vi "Main.vi"() -> ()   [LabVIEW 2015]
doc: "Use this template to build a simple state machine design pattern. Each state executes code and determines which state to transition to."
uses:
  controls/State.ctl
  controls/Data.ctl
  <vilib>/measure/NI_MABase.lvlib
panel:
  in  "Dateiname":string
  out "Waveform Chart":waveform(dbl)(graph)
  in  "Daten speichern":bool
  in  "Signal generieren":bool
  in  "Exit":bool
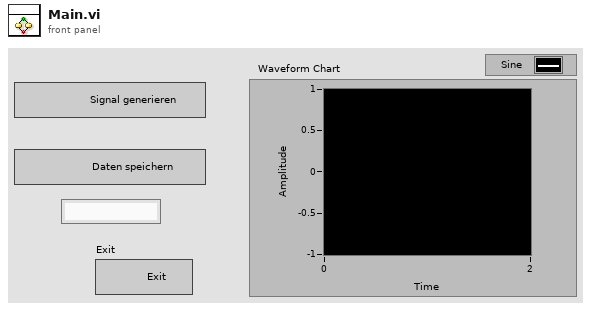
[diagram p1: front panel]
types:
  T1 = typedef "Data.ctl" = cluster{"Boolean":bool, "String":string, "Numeric":dbl, "Waveform":waveform(dbl)}
  T2 = typedef "State.ctl" = enum16{"Initialize", "Wait for Event", "Signal generieren", "Daten speichern", "Exit"}
  T3 = enum16{"open", "open or create", "create or replace", "create", "open (read-only)"}
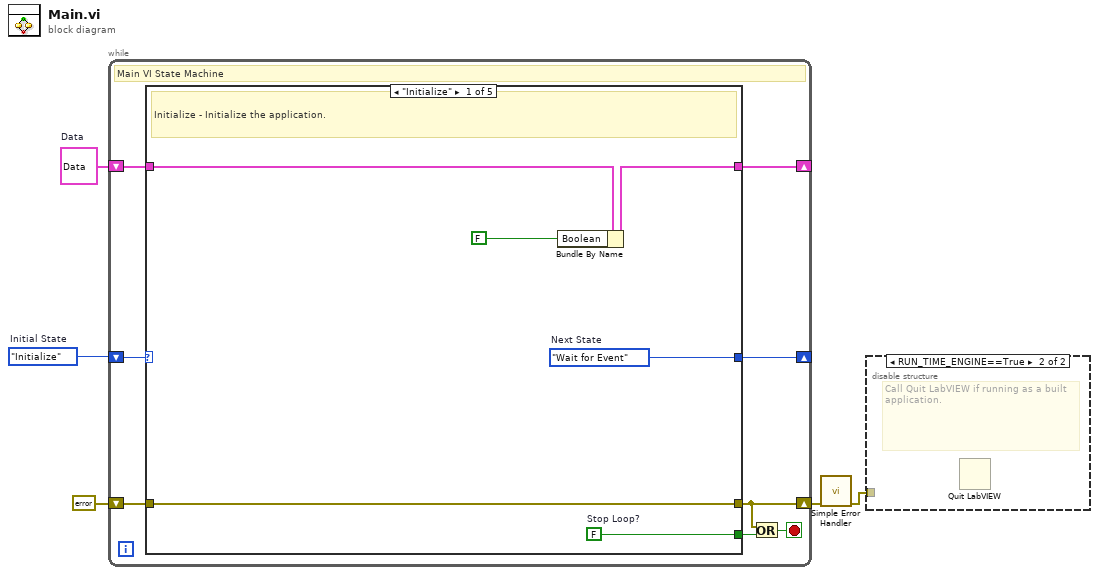
[diagram p0: block diagram]
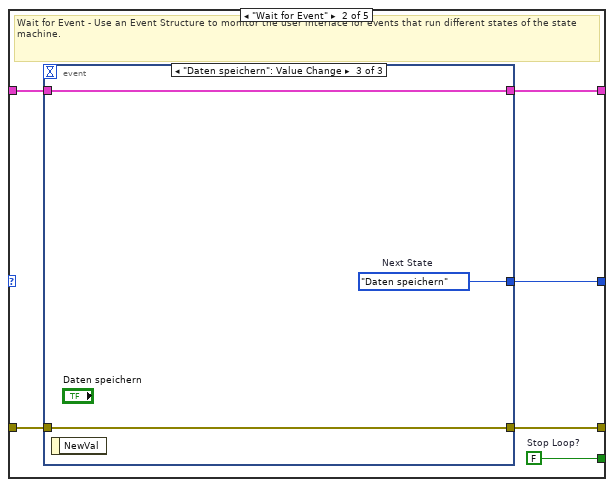
[diagram p3: hidden frame]
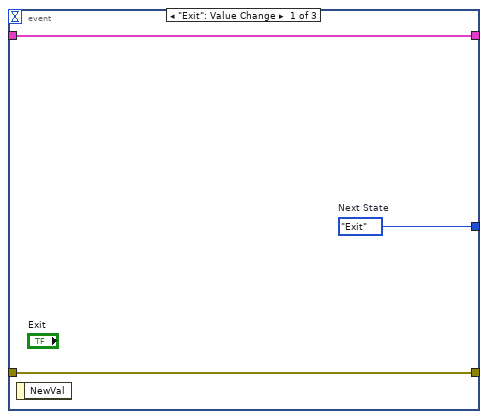
[diagram p4: hidden frame]
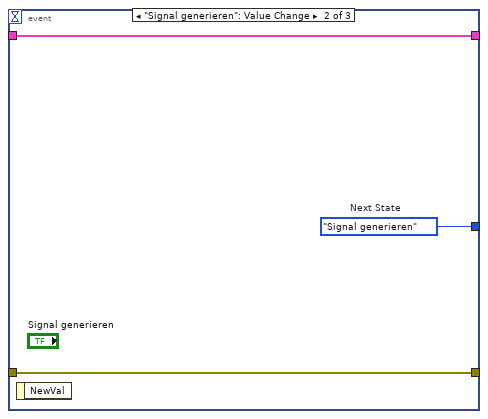
[diagram p5: hidden frame]
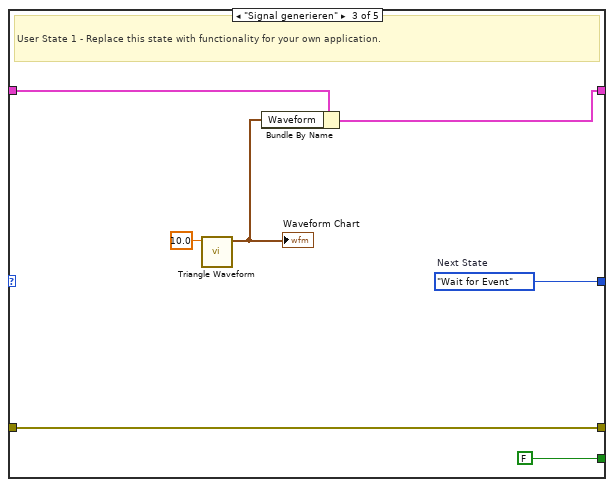
[diagram p6: hidden frame]
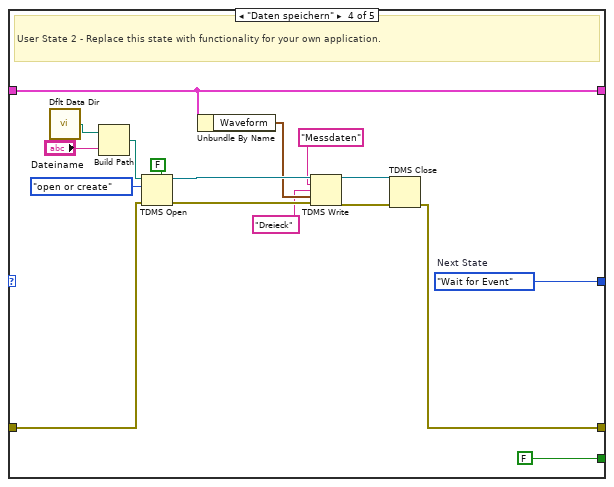
[diagram p7: hidden frame]
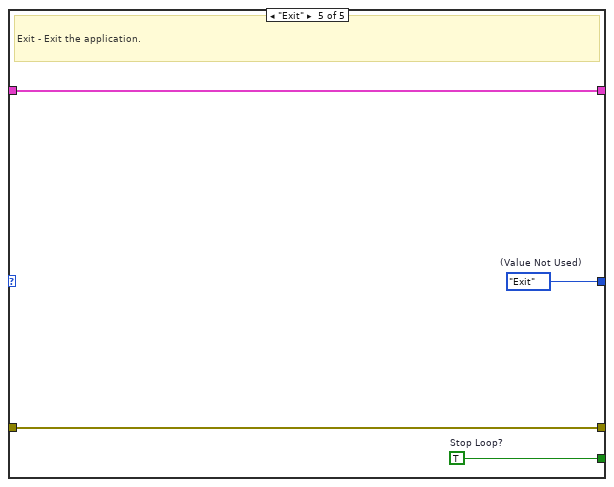
[diagram p8: hidden frame]
diagram:
  w4 = T1 {"Boolean"=FALSE, "String"="", "Numeric"=0.0, "Waveform"={"t0"=timestamp(0 s since 1904-01-01), "dt"=1.0, "Y"=[]}}  # Data
  w5 = State."Initialize"  # Initial State
  n1 = while {
    shift-right: [w12] -> _
    shift-left: w5 -> [w13]
    shift-right: [w10] -> _
    shift-left: w4 -> [w11]
    shift-right: [w6] -> w2
    shift-left: errorcluster {"status"=FALSE, "code"=0, "source"=""} ("error constant") -> [w9]
    stop <- w7 stop-if-true
    # "Main VI State Machine"
    n2 = case shown="\"Initialize\"" w13 {
      tunnel: [w19 w25 w41 w58 w62] -> w12
      tunnel: [w18 w24 FALSE ("Stop Loop?") FALSE ("Stop Loop?") w60] -> w8
      tunnel: w11 -> [w17 w23 w37 w45 w61]
      tunnel: [w16 w22 w36 w45 w61] -> w10
      tunnel: w9 -> [w14 w21 w39 w56 w59]
      tunnel: [w14 w20 w39 w47 w59] -> w6
      frame "Initialize" {
        w18 = FALSE  # Stop Loop?
        w19 = State."Wait for Event"  # Next State
        # "Initialize - Initialize the application."
        n3 = Bundle By Name(cluster=w17, "Boolean"=FALSE ("Replace_Me_Boolean")) -> (w16:T1)
      }
      frame "Wait for Event" {
        w24 = FALSE  # Stop Loop?
        # "Wait for Event - Use an Event Structure to monitor the user interface for events that run different states of the state machine."
        n4 = event shown="[2] \"Daten speichern\": Value Change" {
          selector: _ -> [_ _ _]
          dyn-events: _ -> [_ _ _]
          timeout: _ -> [_ _ _]
          tunnel: [w28 w31 w34] -> w25
          tunnel: w23 -> [w27 w30 w33]
          tunnel: [w27 w30 w33] -> w22
          tunnel: w21 -> [w26 w29 w32]
          tunnel: [w26 w29 w32] -> w20
          event "Exit": Value Change {
            w28 = State."Exit"  # Next State
            n5 = event-data() -> ()  [unwired: 1 in, 1 out]
          }
          event "Signal generieren": Value Change {
            w31 = State."Signal generieren"  # Next State
            n6 = event-data() -> ()  [unwired: 1 in, 1 out]
          }
          event "Daten speichern": Value Change {
            w34 = State."Daten speichern"  # Next State
            n7 = event-data() -> ()  [unwired: 1 in, 1 out]
          }
        }
      }
      frame "Signal generieren" {
        w41 = State."Wait for Event"  # Next State
        # "User State 1 - Replace this state with functionality for your own application."
        n8 = call <vilib>:"Triangle Waveform.vi"("frequency"=10.0) -> ("signal out"=w35:waveform(dbl))  [unwired: 9 in, 1 out]
        "Waveform Chart" <- w35
        n9 = Bundle By Name(cluster=w37, "Waveform"=w35) -> (w36:T1)
      }
      frame "Daten speichern" {
        w58 = State."Wait for Event"  # Next State
        # "User State 2 - Replace this state with functionality for your own application."
        n10 = call <vilib>:"Dflt Data Dir.vi"() -> ("App:Default Data Directory"=w52:path)
        n11 = Build Path(base path=w52, name or relative path="Dateiname") -> (appended path=w54:path)
        n12 = TDMS Open(5:FALSE ("create index file? (T)"), 8:w56, 10:T3."open or create" ("operation (0:open)"), 11:w54) -> (0:w49:errorcluster, 3:w50:refnum<k34>)  [unwired: 3 in]
        n13 = Unbundle By Name(w45) -> ("Waveform"=w44:waveform(dbl))
        n14 = TDMS Write(0:w50, 5:"Messdaten" ("group name in (Untitled)"), 7:"Dreieck" ("channel name(s) in (Untitled)"), 9:w44, 11:w49) -> (4:w46:refnum<k34>, 15:w48:errorcluster)  [unwired: 1 in, 2 out]
        n15 = TDMS Close(8:w48, 11:w46) -> (0:w47:errorcluster)  [unwired: 1 out]
      }
      frame "Exit" {
        w60 = TRUE  # Stop Loop?
        w62 = State."Exit"  # (Value Not Used)
        # "Exit - Exit the application."
      }
    }
    n16 = Or(x=w6, y=w8) -> (x .or. y?=w7:bool)
  }
  n17 = call <vilib>:"Simple Error Handler.vi"("error in (no error)"=w2) -> ("error out"=w1:errorcluster)  [unwired: 4 in, 4 out]
  n18 = disable-structure shown="RUN_TIME_ENGINE==True" {
    disable-tunnel: w1 -> [_ _]
    frame condition #0 (active) {
    }
    frame condition #1 {
      # "Call Quit LabVIEW if running as a built application."
      n19 = Quit LabVIEW() -> ()  [unwired: 1 in]
    }
  }
